vi "FTW-SQLite-Core-LibraryReturnValue.vi"(0 "error in":errorcluster, 7 "Return Value":i32) -> (4 "error out":errorcluster)   [LabVIEW 2014]
uses:
  error/FTW-ERR-ThrowGenericError.vi
  error/FTW-ERR-NoErrorConstant.vi
  error/FTW-ERR-CallChain.vi
  string/FTW-STR-ReplaceWhitespace.vi
panel:
  # "Inputs"
  # "Outputs"
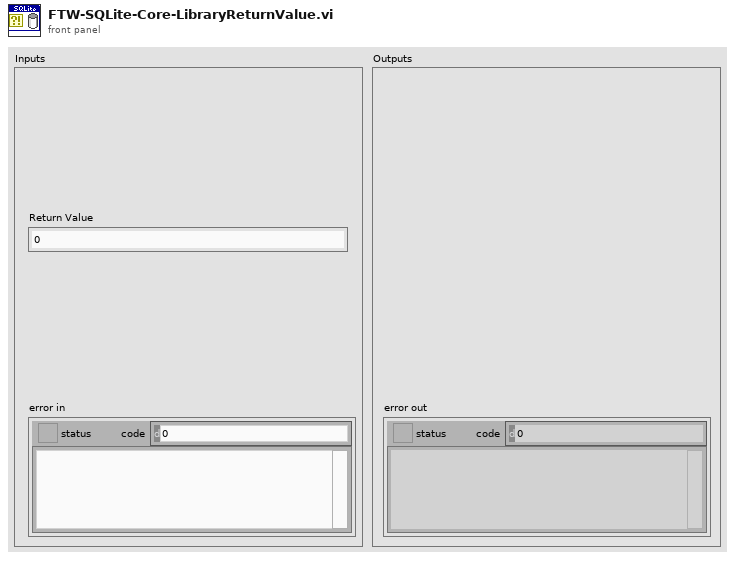
[diagram p1: front panel]
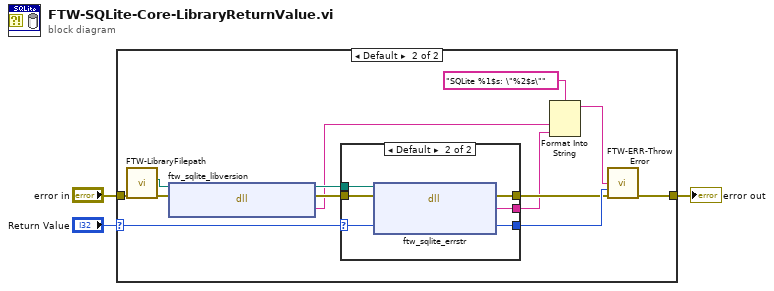
[diagram p0: block diagram]
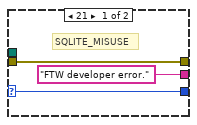
[diagram p3: hidden frame]
diagram:
  n1 = case shown="Default" "Return Value" {
    selector: "Return Value" -> [_ w10]
    tunnel: "error in" -> [w4 w17]
    tunnel: [w4 w16] -> w2
    frame 0 {
    }
    frame Default {
      n2 = call "FTW-LibraryFilepath.vi"("error in"=w17) -> ("error out"=w8:errorcluster, "Library Filepath"=w7:path)  [unwired: 8 in, 1 out]
      n3 = dll-call lib="?" fn="ftw_sqlite_libversion"(path in=w7, error in=w8) -> (path out=w9:path, error out=w6:errorcluster, "Return Value"=w5:string)  [unwired: 1 in]
      n4 = case shown="Default" w10 {
        selector: w10 -> [w20 w21]
        tunnel: w6 -> [w19 w26]
        tunnel: [w20 w25] -> w13
        tunnel: [w19 w24] -> w12
        tunnel: ["FTW developer error." ("Error Message") w23] -> w11
        tunnel: w9 -> [_ w22]
        frame 21 {
          # "SQLITE_MISUSE"
        }
        frame Default {
          n5 = dll-call lib="?" fn="ftw_sqlite_errstr"(path in=w22, error in=w26, "Error Code"=w21) -> (error out=w24:errorcluster, "Error Message"=w23:string, "Error Code"=w25:i32)  [unwired: 1 in, 1 out]
        }
      }
      n6 = Format Into String(format string="SQLite %1$s: \"%2$s\"" ("Error Message"), w5, w11) -> (resulting string=w14:string)  [unwired: 2 in, 1 out]
      n7 = call "FTW-ERR-ThrowError.vi"("Error Message"=w14, "Error Code"=w13, "error in"=w12) -> ("error out"=w16:errorcluster)  [unwired: 12 in]
    }
  }
  "error out" <- w2
